vi "PrepareDevices.vi"() -> ()   [LabVIEW 2010]
uses:
  Controls/Device.ctl
panel:
  out "Devices":T1[](array[typedef])
  in  "Device name":string="HiSPARC III Master A"
  in  "Devices":T1[](array[typedef])
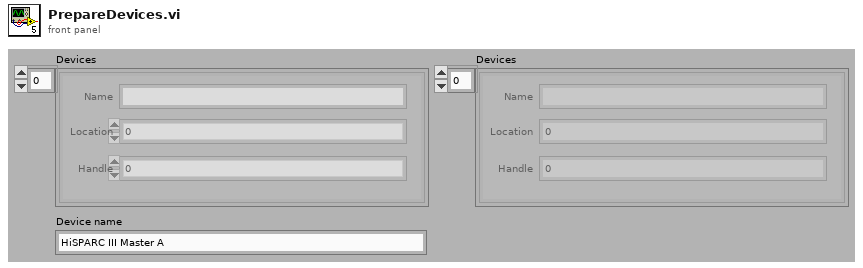
[diagram p1: front panel]
types:
  T1 = typedef "Device.ctl" = cluster{"Name":string, "Location":u32, "Handle":u32}
  T2 = cluster{"GPIOH1 (ACBUS0) I/O":bool, "GPIOH1 (ACBUS0) Hi/Lo":bool, "GPIOH2 (ACBUS1) I/O":bool, "GPIOH2 (ACBUS1) Hi/Lo":bool, "GPIOH3 (ACBUS2) I/O":bool, "GPIOH3 (ACBUS2) Hi/Lo":bool, "GPIOH4 (ACBUS3) I/O":bool, "GPIOH4 (ACBUS3) Hi/Lo":bool}
  T3 = cluster{"CS (ADBUS3)":bool, "GPIOL1 (ADBUS4)":bool, "GPIOL2 (ADBUS5)":bool, "GPIOL3 (ADBUS6)":bool, "GPIOL4 (ADBUS7)":bool}
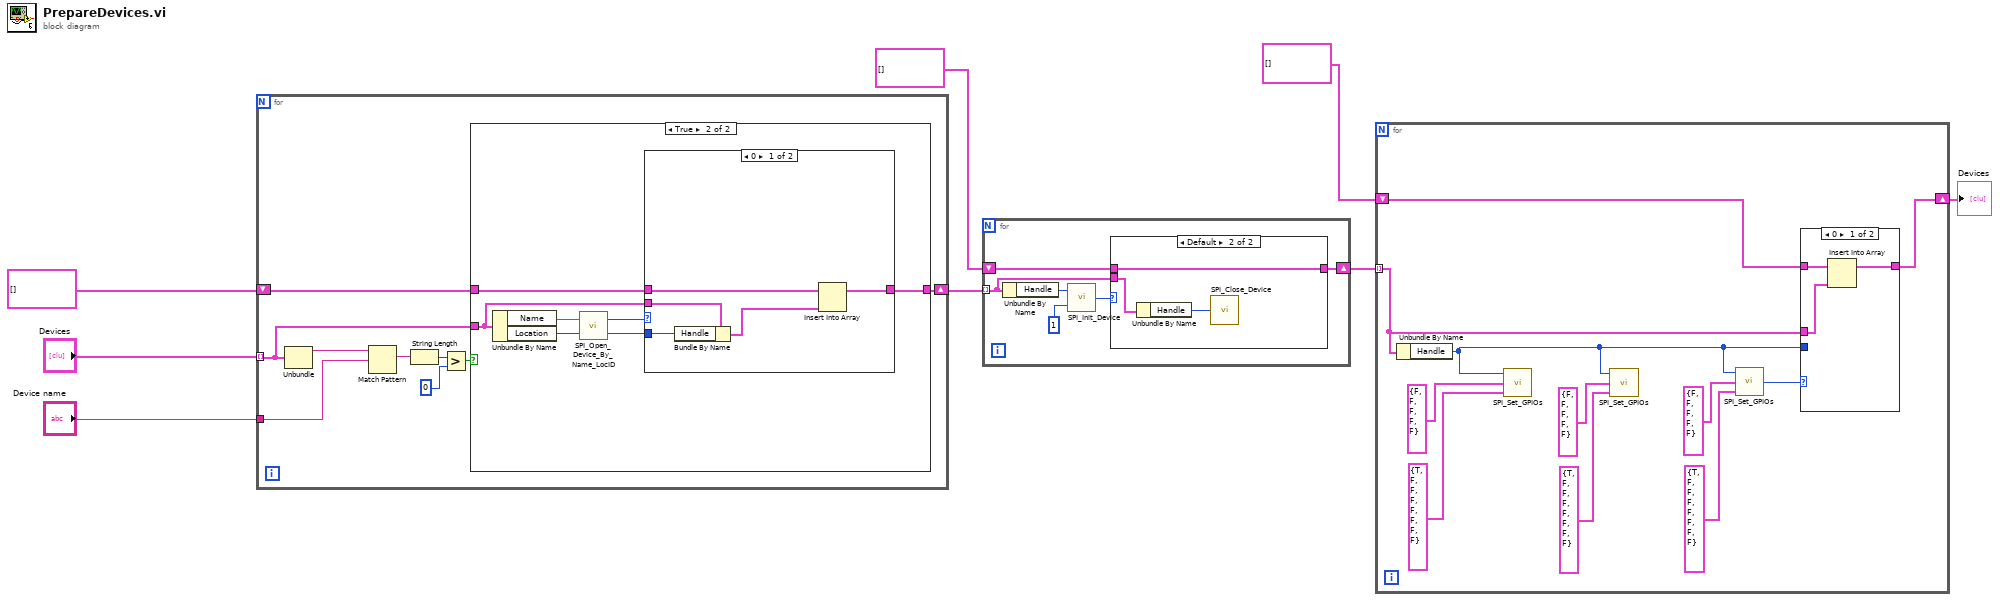
[diagram p0: block diagram]
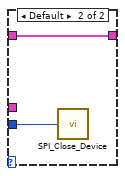
[diagram p2: hidden frame]
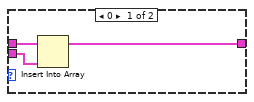
[diagram p3: hidden frame]
diagram:
  n1 = for {
    shift-right: [w9] -> w5
    shift-left: T1[] [] ("Devices 2") -> [w10]
    tunnel: "Devices" -> [w11] mode=indexing
    tunnel: "Device name" -> [w16]
    n2 = Unbundle(w11) -> ("Name"=w17:string)  [unwired: 2 out]
    n3 = Match Pattern(string=w17, regular expression=w16) -> (match substring=w15:string)  [unwired: 1 in, 3 out]
    n4 = String Length(string=w15) -> (length=w13:i32)
    n5 = Greater?(x=w13, y=0) -> (0:w14:bool)
    n6 = case shown="True" w14 {
      tunnel: w11 -> [_ w19]
      tunnel: w10 -> [w18 w21]
      tunnel: [w18 w22] -> w9
      frame False {
      }
      frame True {
        n7 = Unbundle By Name(w19) -> ("Name"=w25:string, "Location"=w24:u32)
        n8 = call "SPI_Open_Device_By_Name_LocID.vi"("LocID"=w24, "DeviceName"=w25) -> ("Handle"=w20:u32, "FTC_Status"=w23:u32)
        n9 = case shown="0" w23 {
          tunnel: [w26 w31] -> w22
          tunnel: w21 -> [w30 w31]
          tunnel: w20 -> [w28 _]
          tunnel: w19 -> [w29 _]
          frame 0 {
            n10 = Bundle By Name(cluster=w29, "Handle"=w28) -> (w27:T1)
            n11 = Insert Into Array(array=w30, new element=w27) -> (w26:T1[])  [unwired: 1 in]
          }
          frame Default {
          }
        }
      }
    }
  }
  n12 = for {
    tunnel: w5 -> [w32] mode=indexing
    shift-right: [w33] -> w3
    shift-left: T1[] [] ("Devices 2") -> [w34]
    n13 = Unbundle By Name(w32) -> ("Handle"=w37:u32)
    n14 = call "SPI_Init_Device.vi"("ClockDivisor"=u32 1, "Handle"=w37) -> ("FTC_Status"=w35:u32)
    n15 = case shown="Default" w35 {
      tunnel: w34 -> [w40 w43]
      tunnel: [w38 w43] -> w33
      tunnel: w32 -> [w39 w42]
      frame 0 {
        n16 = Insert Into Array(array=w40, new element=w39) -> (w38:T1[])  [unwired: 1 in]
      }
      frame Default {
        n17 = Unbundle By Name(w42) -> ("Handle"=w41:u32)
        n18 = call "SPI_Close_Device.vi"("Handle"=w41) -> ()  [unwired: 1 out]
      }
    }
  }
  n19 = for {
    tunnel: w3 -> [w45] mode=indexing
    shift-right: [w46] -> w1
    shift-left: T1[] [] ("Devices 2") -> [w47]
    n20 = Unbundle By Name(w45) -> ("Handle"=w44:u32)
    n21 = call "SPI_Set_GPIOs.vi"("High IOs Config"=T2 {"GPIOH1 (ACBUS0) I/O"=TRUE, "GPIOH1 (ACBUS0) Hi/Lo"=FALSE, "GPIOH2 (ACBUS1) I/O"=FALSE, "GPIOH2 (ACBUS1) Hi/Lo"=FALSE, "GPIOH3 (ACBUS2) I/O"=FALSE, "GPIOH3 (ACBUS2) Hi/Lo"=FALSE, "GPIOH4 (ACBUS3) I/O"=FALSE, "GPIOH4 (ACBUS3) Hi/Lo"=FALSE}, "CSDisableStates"=T3 {"CS (ADBUS3)"=FALSE, "GPIOL1 (ADBUS4)"=FALSE, "GPIOL2 (ADBUS5)"=FALSE, "GPIOL3 (ADBUS6)"=FALSE, "GPIOL4 (ADBUS7)"=FALSE}, "Handle"=w44) -> ()  [unwired: 1 out]
    n22 = call "SPI_Set_GPIOs.vi"("High IOs Config"=T2 {"GPIOH1 (ACBUS0) I/O"=TRUE, "GPIOH1 (ACBUS0) Hi/Lo"=FALSE, "GPIOH2 (ACBUS1) I/O"=FALSE, "GPIOH2 (ACBUS1) Hi/Lo"=FALSE, "GPIOH3 (ACBUS2) I/O"=FALSE, "GPIOH3 (ACBUS2) Hi/Lo"=FALSE, "GPIOH4 (ACBUS3) I/O"=FALSE, "GPIOH4 (ACBUS3) Hi/Lo"=FALSE}, "CSDisableStates"=T3 {"CS (ADBUS3)"=FALSE, "GPIOL1 (ADBUS4)"=FALSE, "GPIOL2 (ADBUS5)"=FALSE, "GPIOL3 (ADBUS6)"=FALSE, "GPIOL4 (ADBUS7)"=FALSE}, "Handle"=w44) -> ()  [unwired: 1 out]
    n23 = call "SPI_Set_GPIOs.vi"("High IOs Config"=T2 {"GPIOH1 (ACBUS0) I/O"=TRUE, "GPIOH1 (ACBUS0) Hi/Lo"=FALSE, "GPIOH2 (ACBUS1) I/O"=FALSE, "GPIOH2 (ACBUS1) Hi/Lo"=FALSE, "GPIOH3 (ACBUS2) I/O"=FALSE, "GPIOH3 (ACBUS2) Hi/Lo"=FALSE, "GPIOH4 (ACBUS3) I/O"=FALSE, "GPIOH4 (ACBUS3) Hi/Lo"=FALSE}, "CSDisableStates"=T3 {"CS (ADBUS3)"=FALSE, "GPIOL1 (ADBUS4)"=FALSE, "GPIOL2 (ADBUS5)"=FALSE, "GPIOL3 (ADBUS6)"=FALSE, "GPIOL4 (ADBUS7)"=FALSE}, "Handle"=w44) -> ("FTC_Status"=w48:u32)
    n24 = case shown="0" w48 {
      tunnel: w47 -> [w57 w59]
      tunnel: [w56 w59] -> w46
      tunnel: w45 -> [w55 _]
      tunnel: w44 -> [_ w58]
      frame 0 {
        n25 = Insert Into Array(array=w57, new element=w55) -> (w56:T1[])  [unwired: 1 in]
      }
      frame Default {
        n26 = call "SPI_Close_Device.vi"("Handle"=w58) -> ()  [unwired: 1 out]
      }
    }
  }
  "Devices" <- w1
